vi "NewTest.vi"(8 "error in (no error)":errorcluster, 10 "NewTest":T1, 11 "UnitTestEngine in":refnum<class "UnitTestEngine.lvclass">) -> (0 "error out":errorcluster, 3 "UnitTestEngine out":refnum<class "UnitTestEngine.lvclass">)   [LabVIEW 2019, in "UnitTestEngine.lvlib" / "UnitTestEngine.lvclass"]
uses:
  UnitTestEngine.lvclass
  <vilib>/Utility/miscctls.llb/LVRowAndColumnUnsignedTypeDef.ctl
  <vilib>/Utility/miscctls.llb/LVRowAndColumnTypeDef.ctl
  UnitTestEngine.lvclass/UnitTestEngine.ctl
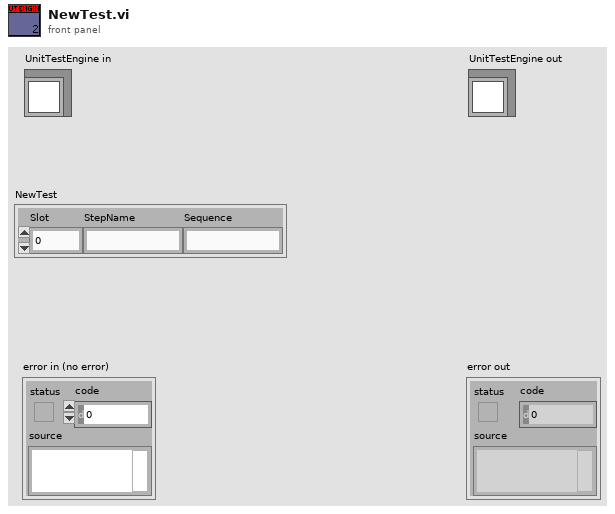
[diagram p1: front panel]
types:
  T1 = cluster{"Slot":i32, "StepName":string, "Sequence":string}
  T2 = typedef "LVRowAndColumnTypeDef.ctl" = cluster{"Row":i32, "Column":i32}
  T3 = typedef "LVRowAndColumnUnsignedTypeDef.ctl" = cluster{"Row":u32, "Column":u32}
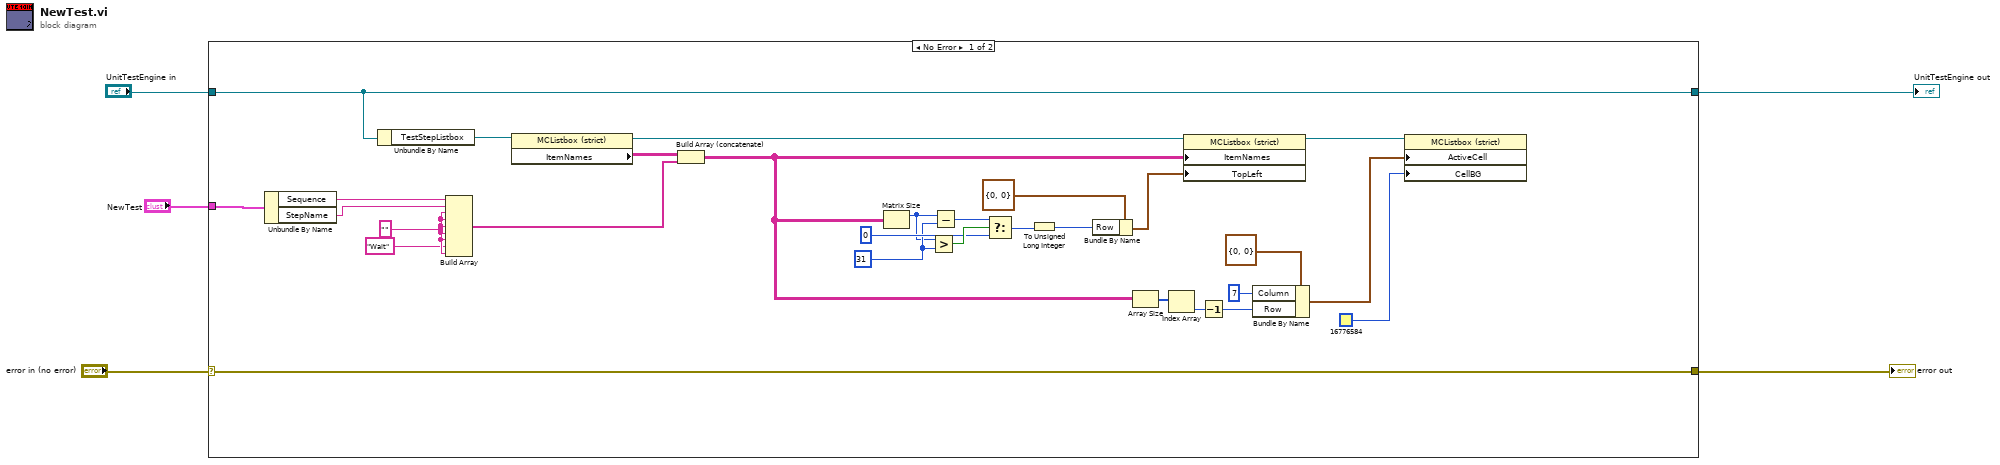
[diagram p0: block diagram]
diagram:
  n1 = case shown="No Error" "error in (no error)" {
    selector: "error in (no error)" -> [w34 w36]
    tunnel: [w34 w36] -> w4
    tunnel: [w32 w35] -> w2
    tunnel: "UnitTestEngine in" -> [w32 w35]
    tunnel: "NewTest" -> [w33 _]
    frame No Error {
      w17 = 31
      w28 = "" ("element")
      n2 = Unbundle By Name(w33) -> ("Sequence"=w29:string, "StepName"=w6:string)
      n3 = Unbundle By Name(w32) -> ("TestStepListbox"=w31:refnum<vi>)
      n4 = Build Array(w29, w6, w28, w28, w28, w28, w28, "Wait" ("element"), w28) -> (w26:string[])
      n5 = property class="MCListbox (strict)"(reference=w31) -> (reference out=w13:refnum<vi>, "ItemNames"=w30:string[][])  [unwired: 1 in, 1 out]
      n6 = Build Array (concatenate)(w30, w26) -> (w14:string[][])
      n7 = Matrix Size(0:w14) -> (1:w16:i32)  [unwired: 1 out]
      n8 = Greater?(x=w16, y=w17) -> (0:w22:bool)
      n9 = Subtract(x=w16, y=w17) -> (x-y=w20:i32)
      n10 = Select(t=w20, s=w22, f=0) -> (s? t:f=w19:i32)
      n11 = To Unsigned Long Integer(number=w19) -> (unsigned 32bit integer=w23:u32)
      n12 = Bundle By Name(cluster=T3 {"Row"=0, "Column"=0} ("Top Left Visible Cell"), "Row"=w23) -> (w15:T3)
      n13 = Array Size(array=w14) -> (size(s)=w10:i32[])
      n14 = Index Array(array=w10) -> (element=w9:i32)  [unwired: 1 in]
      n15 = property class="MCListbox (strict)"(reference=w13, "ItemNames"=w14, "TopLeft"=w15) -> (reference out=w25:refnum<vi>)  [unwired: 1 in, 1 out]
      n16 = Decrement(x=w9) -> (x-1=w8:i32)
      n17 = Bundle By Name(cluster=T2 {"Row"=0, "Column"=0} ("Active Cell:Active Cell"), "Column"=7, "Row"=w8) -> (w24:T2)
      n18 = property class="MCListbox (strict)"(reference=w25, "ActiveCell"=w24, "CellBG"=u32 16776584 ("Text.Text Colors:Text Color")) -> ()  [unwired: 1 in, 2 out]
    }
    frame Error {
    }
  }
  "error out" <- w4
  "UnitTestEngine out" <- w2
